vi "Add To DAQmx Task.vi"(6 "Ignore Cal? (F)":bool, 7 "Tachometer in":refnum<class "Tachometer.lvclass">, 8 "error in (no error)":errorcluster, 9 "Scale Name":string, 10 "Chassis Name":string, 11 "task in":refnum<k21>) -> (0 "error out":errorcluster, 2 "Phys Chan Added":string, 3 "task out":refnum<k21>)   [LabVIEW 2012, in "Measurement Channels.lvlib" / "Tachometer.lvclass"]
uses:
  Tachometer.lvclass
  Class Frequency/Frequency.lvclass
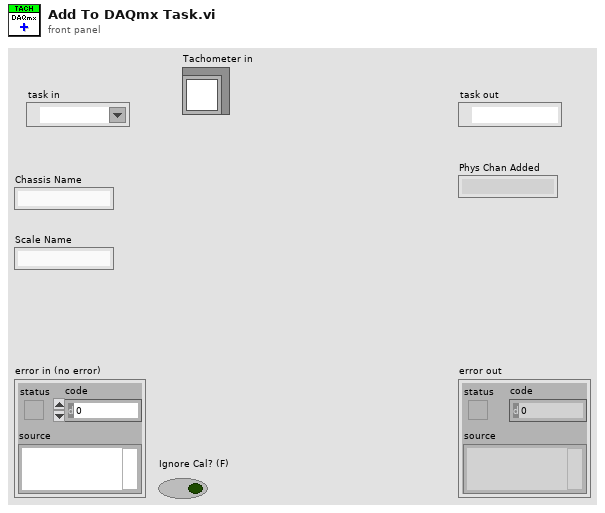
[diagram p1: front panel]
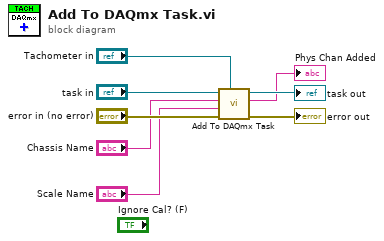
[diagram p0: block diagram]
diagram:
  n1 = call-parent "Add To DAQmx Task.vi"("Frequency in"="Tachometer in", "error in (no error)"="error in (no error)", "Scale Name"="Scale Name", "Chassis Name"="Chassis Name", "task in"="task in") -> ("error out"=→"error out":errorcluster, "Phys Chan Added"=→"Phys Chan Added":string, "task out"=→"task out":refnum<k21>)  [unwired: 4 in]
